vi "StdsWaveforms.vi"() -> (0 "Std 1D Array":dbl[][](array[numeric]), 1 "Table":string[][](table), 3 "Stds Chart":dbl(graph))   [LabVIEW 2023]
panel:
  out "Waveform Graph":dbl[][](graph)
  out "All Results":dbl[][](array[numeric])
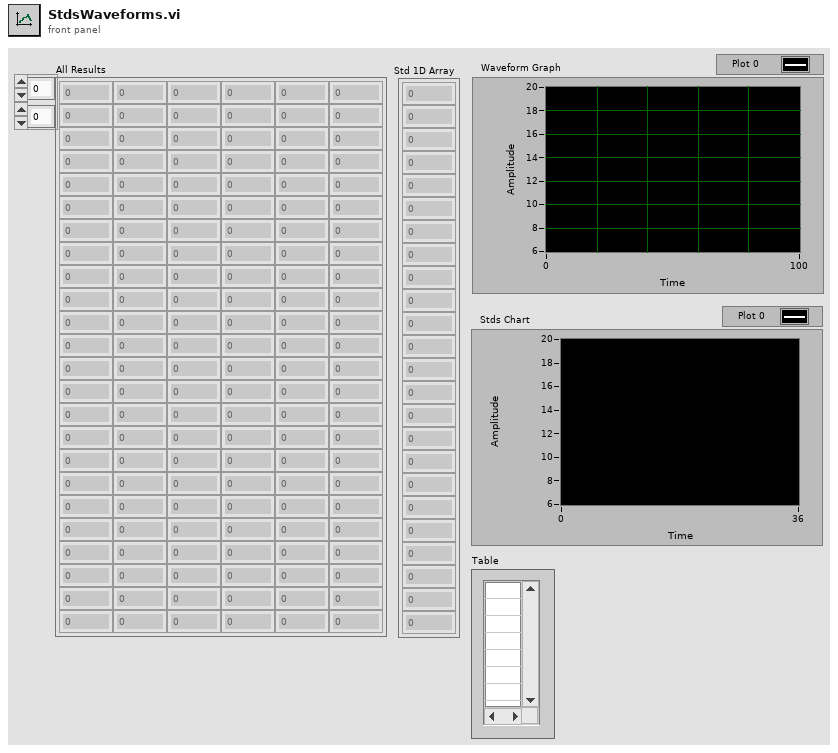
[diagram p1: front panel]
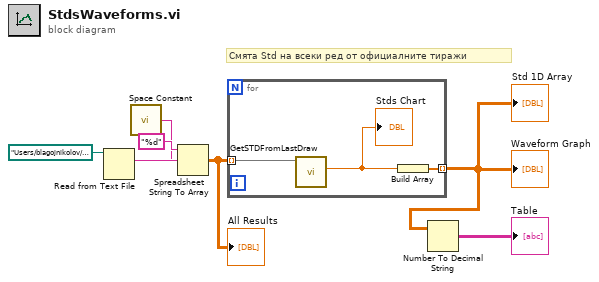
[diagram p0: block diagram]
diagram:
  # "Смята Std на всеки ред от официалните тиражи"
  n1 = Read from Text File(file (use dialog)=path "/Users/blagojnikolov/Desktop/@tmp/results.txt") -> (text=w6:string)  [unwired: 3 in, 3 out]
  n2 = call <vilib>:"Space Constant.vi"() -> ("String"=w4:string)
  n3 = Spreadsheet String To Array(delimiter (Tab)=w4, format string="%d", spreadsheet string=w6) -> (array=w3:dbl[][])  [unwired: 1 in]
  "All Results" <- w3
  n4 = for {
    tunnel: w3 -> [w9] mode=indexing
    tunnel: [w10] -> w2 mode=indexing
    n5 = call "GetSTDFromLastDraw.vi"("Officials Results"=w9) -> ("STD"=w8:dbl)  [unwired: 8 in, 2 out]
    "Stds Chart" <- w8
    n6 = Build Array(w8) -> (w10:dbl[])
  }
  "Std 1D Array" <- w2
  "Waveform Graph" <- w2
  n7 = Number To Decimal String(number=w2) -> (decimal integer string=→"Table":string[][])  [unwired: 1 in]
